vi "_Parse IEM Margin Segment Result.vi"(8 "error in (no error)":errorcluster, 10 "Input String":string, 11 "VISA resource name":refnum<visa-resource-name>) -> (0 "error out":errorcluster, 1 "IEM Margin Results":T2 {"Carrier Leakage" format="%^.3e"; "IQ Image" format="%^.3e"; "General" format="%^.3e"}, 2 "Reliability Results":T1, 3 "VISA resource name out":refnum<visa-resource-name>, 5 "Out Of Tolerance":dbl format="%^.3e", 7 "Statistic Expired":i32)   [LabVIEW 2020, in "Rohde&Schwarz CMWXP NR FR1 Measurement.lvlib"]
uses:
  <instrlib>/Rohde&Schwarz CMWXP NR FR1 Measurement/Rohde&Schwarz CMWXP NR FR1 Measurement.lvlib
  <instrlib>/Rohde&Schwarz CMWXP NR FR1 Measurement/Private/rsidr_core.llb/rsidr_core.lvlib
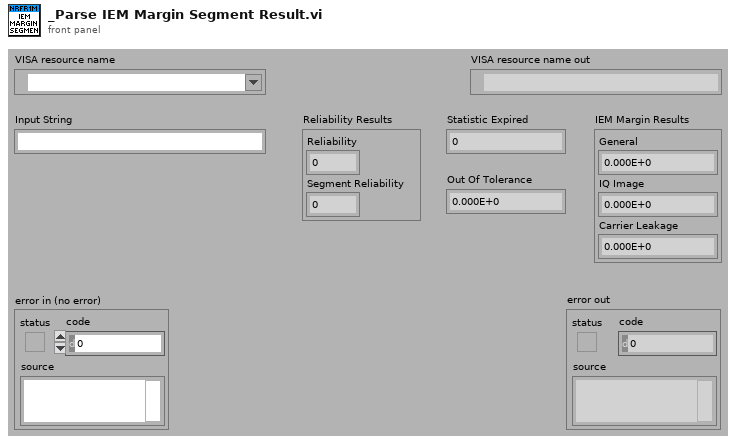
[diagram p1: front panel]
types:
  T1 = cluster{"Reliability":i32, "Segment Reliability":i32}
  T2 = cluster{"General":dbl, "IQ Image":dbl, "Carrier Leakage":dbl}
  T3 = typedef "Rohde&Schwarz CMWXP NR FR1 Measurement.lvlib/_SegReliability.ctl" = cluster{"Reliability":i32, "Segment Reliability":i32}
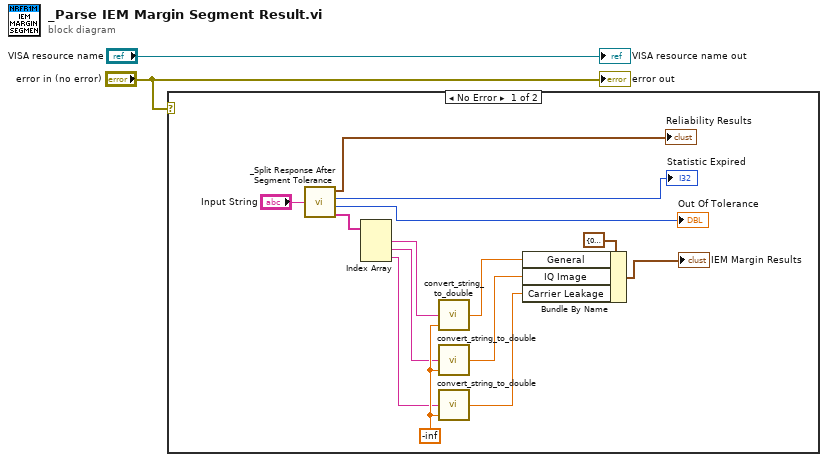
[diagram p0: block diagram]
diagram:
  n1 = case shown="No Error" "error in (no error)" {
    frame No Error {
      w12 = -inf
      n2 = call <instrlib>:"_Split Response After Segment Tolerance.vi"("Input String"="Input String") -> ("Reliability Results"=→"Reliability Results":T3, "Statistic Expired"=→"Statistic Expired":i32, "Out Of Tolerance"=→"Out Of Tolerance":i32, "Response out"=w14:string[])
      n3 = Index Array(array=w14) -> (element #1=w13:string, element #2=w9:string, element #3=w10:string)  [unwired: 3 in]
      n4 = call <instrlib>:"convert_string_to_double.vi"("default (0)"=w12, "String in"=w13) -> ("double value out"=w16:dbl)  [unwired: 3 in]
      n5 = call <instrlib>:"convert_string_to_double.vi"("default (0)"=w12, "String in"=w9) -> ("double value out"=w8:dbl)  [unwired: 3 in]
      n6 = call <instrlib>:"convert_string_to_double.vi"("default (0)"=w12, "String in"=w10) -> ("double value out"=w11:dbl)  [unwired: 3 in]
      n7 = Bundle By Name(cluster=T2 {"General"=0.0, "IQ Image"=0.0, "Carrier Leakage"=0.0} ("IEM Margin Results"), "General"=w16, "IQ Image"=w8, "Carrier Leakage"=w11) -> (→"IEM Margin Results":T2)
    }
    frame Error {
    }
  }
  "error out" <- "error in (no error)"
  "VISA resource name out" <- "VISA resource name"
